vi "PrimeNumberCalculator.vi"() -> ()   [LabVIEW 2020]
panel:
  out "Result":string
  in  "N":i32
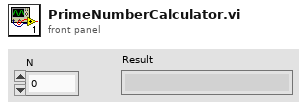
[diagram p1: front panel]
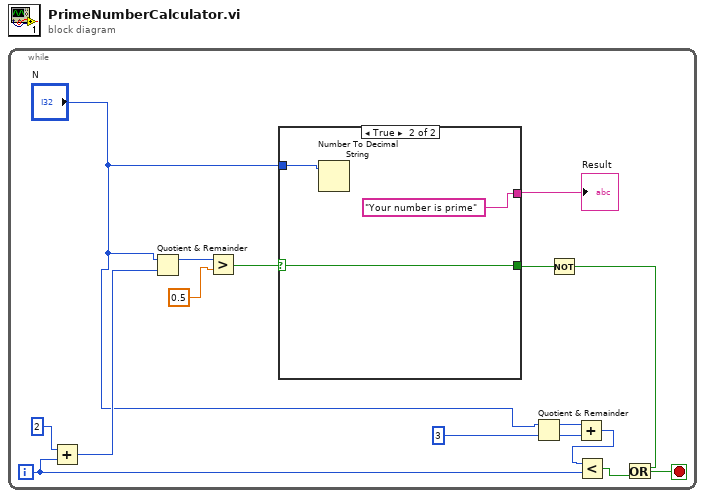
[diagram p0: block diagram]
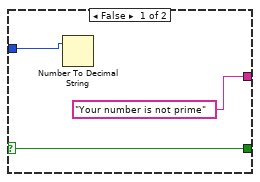
[diagram p2: hidden frame]
diagram:
  n1 = while {
    i -> [w12]
    stop <- w4 stop-if-true
    n2 = Add(x=2, y=w12) -> (x+y=w11:i32)
    n3 = Quotient & Remainder(x="N", y=w11) -> (x-y*floor(x/y)=w10:i32)  [unwired: 1 out]
    n4 = Greater?(x=w10, y=0.5) -> (0:w7:bool)
    n5 = case shown="True" w7 {
      selector: w7 -> [w18 w21]
      tunnel: "N" -> [w19 w22]
      tunnel: [w18 w21] -> w6
      tunnel: ["Your number is not prime" "Your number is prime"] -> w1
      frame False {
        n6 = Number To Decimal String(number=w19) -> ()  [unwired: 1 in, 1 out]
      }
      frame True {
        n7 = Number To Decimal String(number=w22) -> ()  [unwired: 1 in, 1 out]
      }
    }
    "Result" <- w1
    n8 = Quotient & Remainder(x="N", y=3) -> (x-y*floor(x/y)=w14:i32, floor(x/y)=w15:i32)
    n9 = Not(x=w6) -> (.not. x?=w2:bool)
    n10 = Add(x=w14, y=w15) -> (x+y=w5:i32)
    n11 = Less?(x=w5, y=w12) -> (x < y?=w3:bool)
    n12 = Or(x=w2, y=w3) -> (x .or. y?=w4:bool)
  }
